vi "Clear Old Log Folders.vi"(8 "error in (no error)":errorcluster) -> (0 "error out":errorcluster)   [LabVIEW 2020, in "Global_logger.lvlib"]
uses:
  Global_logger.lvlib
  Logger Output.ctl
  Levels.ctl
  Level Meaning.ctl
  Sorting.ctl
  Logger Type.ctl
  Log Fields.ctl
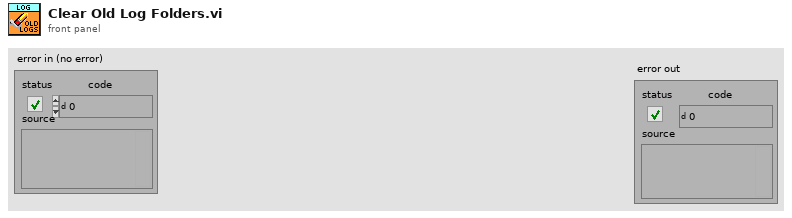
[diagram p1: front panel]
types:
  T1 = typedef "Global_logger.lvlib/Logger Output.ctl" = cluster{"Level":T2, "Level Meaning":T3, "Sorting":T4, "Type":T5, "Filetype":string, "Filename":string, "Root path":path, "Max filesize (bytes)":i32, "Max age (days)":i32, "Ctl Refnum":refnum<vi>, "String Ctl Delimiter":string, "Format":T6[], "Timestamp format":string}
  T2 = typedef "Global_logger.lvlib/Levels.ctl" = enum16{"ALL", "TRACE", "DEBUG", "INFO", "WARN", "ERROR", "FATAL", "OFF"}
  T3 = typedef "Global_logger.lvlib/Level Meaning.ctl" = enum16{"Standard", "Positive", "Exact"}
  T4 = typedef "Global_logger.lvlib/Sorting.ctl" = enum16{"Add to Bottom", "Add to Top"}
  T5 = typedef "Global_logger.lvlib/Logger Type.ctl" = enum16{"FILE", "UI"}
  T6 = typedef "Global_logger.lvlib/Log Fields.ctl" = enum16{"Timestamp", "Level", "Message", "Source VI", "Source App", "Logger Name"}
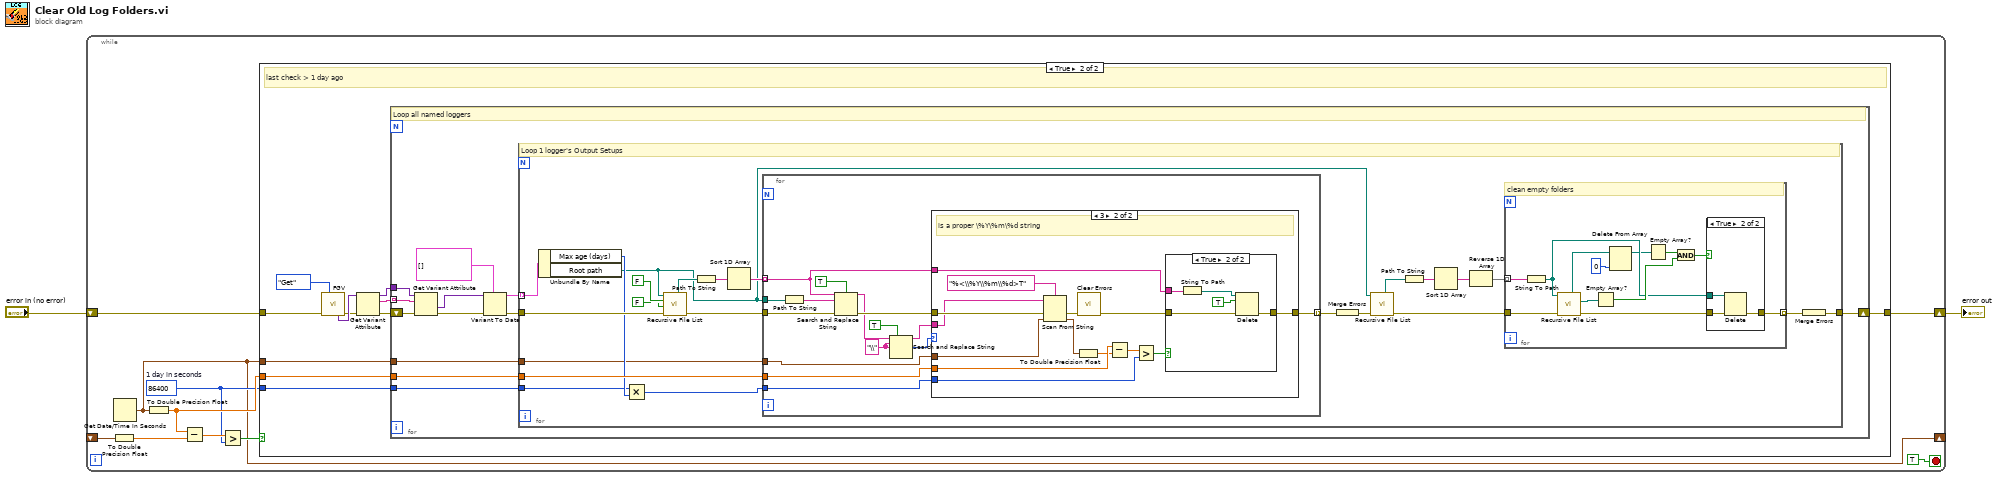
[diagram p0: block diagram]
diagram:
  n1 = while {
    shift-right: [w11] -> w1
    shift-left: "error in (no error)" -> [w12]
    shift-right: [w3] -> _
    shift-left: _ -> [w9]
    stop <- TRUE stop-if-true
    w4 = u32 86400  # 1 day in seconds
    n2 = To Double Precision Float(number=w9) -> (double precision float=w8:dbl)
    n3 = Get Date/Time In Seconds() -> (seconds since 1Jan1904=w3:timestamp)
    n4 = To Double Precision Float(number=w3) -> (double precision float=w5:dbl)
    n5 = Subtract(x=w5, y=w8) -> (x-y=w7:dbl)
    n6 = Greater?(x=w7, y=w4) -> (0:w6:bool)
    n7 = case shown="True" w6 {
      tunnel: w12 -> [w13 w24]
      tunnel: [w13 w19] -> w11
      tunnel: w5 -> [_ w22]
      tunnel: w4 -> [_ w21]
      tunnel: w3 -> [_ w20]
      frame False {
      }
      frame True {
        # "last check > 1 day ago"
        n8 = call "FGV.vi"("Action"=enum16{"Get", "Set"}."Get", "error in (no error)"=w24) -> ("All Named Loggers"=w18:variant, "error out"=w17:errorcluster)  [unwired: 8 in, 4 out]
        n9 = Get Variant Attribute(Variant=w18, error in=w17) -> (duplicate Variant=w14:variant, names=w15:string[], error out=w16:errorcluster)  [unwired: 2 in, 1 out]
        n10 = for {
          tunnel: w22 -> [w36]
          tunnel: w21 -> [w35]
          tunnel: w20 -> [w34]
          shift-right: [w33] -> w19
          shift-left: w16 -> [w27]
          tunnel: w15 -> [w29] mode=indexing
          tunnel: w14 -> [w28]
          # "Loop all named loggers"
          n11 = Get Variant Attribute(Variant=w28, name=w29, error in=w27) -> (value=w25:variant, error out=w26:errorcluster)  [unwired: 1 in, 2 out]
          n12 = Variant To Data(error in=w26, type=T1[] [], Variant=w25) -> (data=w30:T1[], error out=w31:errorcluster)
          n13 = for {
            tunnel: w31 -> [w59]
            tunnel: w36 -> [w52]
            tunnel: w35 -> [w50]
            tunnel: w34 -> [w47]
            tunnel: [w39] -> w33
            tunnel: w30 -> [w38] mode=indexing
            # "Loop 1 logger's Output Setups"
            n14 = Unbundle By Name(w38) -> ("Max age (days)"=w51:i32, "Root path"=w37:path)
            n15 = Multiply(x=w50, y=w51) -> (x*y=w49:u32)
            n16 = call <vilib>:"Recursive File List.vi"("error in (no error)"=w59, "Continue Recursing on Error? (F)"=FALSE, "Treat LLBs as Folders?"=FALSE, "Folder Path"=w37) -> ("error out"=w53:errorcluster, "All Folders"=w56:path[])  [unwired: 3 in, 3 out]
            n17 = Path To String(path=w56) -> (string=w55:string[])
            n18 = Sort 1D Array(array=w55) -> (sorted array=w54:string[])
            n19 = for {
              tunnel: w54 -> [w83] mode=indexing
              tunnel: w37 -> [w85]
              tunnel: w53 -> [w88]
              tunnel: w52 -> [w87]
              tunnel: w49 -> [w86]
              tunnel: [w84] -> w48 mode=indexing
              tunnel: w47 -> [w82]
              w78 = "\\" ("search string")
              n20 = Path To String(path=w85) -> (string=w90:string)
              n21 = Search and Replace String(case sensitive?=TRUE ("ignore case? (F)"), input string=w83, search string=w90, error in=w88) -> (result string=w80:string, error out=w81:errorcluster)  [unwired: 4 in, 2 out]
              n22 = Search and Replace String(replace all?=TRUE ("replace all? (F)"), input string=w80, search string=w78, replace string=w78) -> (result string=w77:string, number of replacements=w76:i32)  [unwired: 4 in, 2 out]
              n23 = case shown="3" w76 {
                tunnel: w87 -> [_ w104]
                tunnel: w86 -> [_ w101]
                tunnel: [w91 w99] -> w84
                tunnel: w83 -> [_ w98]
                tunnel: w82 -> [_ w97]
                tunnel: w81 -> [w91 w93]
                tunnel: w77 -> [_ w92]
                frame 0, Default {
                }
                frame 3 {
                  # "is a proper \\%Y\\%m\\%d string"
                  n24 = Scan From String(format string="%<\\%Y\\%m\\%d>T", input string=w92, error in=w93, default 1=w97) -> (error out=w95:errorcluster, output 1=w96:timestamp)  [unwired: 1 in, 2 out]
                  n25 = To Double Precision Float(number=w96) -> (double precision float=w103:dbl)
                  n26 = call <vilib>:"Clear Errors.vi"("error in (no error)"=w95) -> ("error out"=w94:errorcluster)  [unwired: 5 in, 1 out]
                  n27 = Subtract(x=w104, y=w103) -> (x-y=w102:dbl)
                  n28 = Greater?(x=w102, y=w101) -> (0:w100:bool)
                  n29 = case shown="True" w100 {
                    tunnel: w98 -> [_ w108]
                    tunnel: w94 -> [w106 w111]
                    tunnel: [w106 w110] -> w99
                    frame False {
                    }
                    frame True {
                      n30 = String To Path(string=w108) -> (path=w107:path)
                      n31 = Delete(path (use dialog)=w107, entire hierarchy (F)=TRUE, error in=w111) -> (error out=w110:errorcluster)  [unwired: 2 in, 2 out]
                    }
                  }
                }
              }
            }
            n32 = Merge Errors(w48) -> (w46:errorcluster)
            n33 = call <vilib>:"Recursive File List.vi"("error in (no error)"=w46, "Folder Path"=w37) -> ("error out"=w41:errorcluster, "All Folders"=w44:path[])  [unwired: 5 in, 3 out]
            n34 = Path To String(path=w44) -> (string=w45:string[])
            n35 = Sort 1D Array(array=w45) -> (sorted array=w43:string[])
            n36 = Reverse 1D Array(array=w43) -> (reversed array=w42:string[])
            n37 = for {
              tunnel: w42 -> [w71] mode=indexing
              tunnel: w41 -> [w70]
              tunnel: [w64] -> w40 mode=indexing
              # "clean empty folders"
              n38 = String To Path(string=w71) -> (path=w66:path)
              n39 = call <vilib>:"Recursive File List.vi"("error in (no error)"=w70, "Folder Path"=w66) -> ("error out"=w65:errorcluster, "All Files in Dir"=w69:path[], "All Folders"=w62:path[])  [unwired: 5 in, 2 out]
              n40 = Empty Array?(array=w69) -> (empty?=w67:bool)
              n41 = Delete From Array(array=w62, index=0) -> (array with subset deleted=w61:path[])  [unwired: 1 in, 1 out]
              n42 = Empty Array?(array=w61) -> (empty?=w68:bool)
              n43 = And(x=w68, y=w67) -> (x .and. y?=w63:bool)
              n44 = case shown="True" w63 {
                tunnel: w66 -> [_ w75]
                tunnel: w65 -> [w72 w74]
                tunnel: [w72 w73] -> w64
                frame False {
                }
                frame True {
                  n45 = Delete(path (use dialog)=w75, error in=w74) -> (error out=w73:errorcluster)  [unwired: 3 in, 2 out]
                }
              }
            }
            n46 = Merge Errors(w40) -> (w39:errorcluster)
          }
        }
      }
    }
  }
  "error out" <- w1
